vi "Log in with Email and Password.vi"() -> ()   [LabVIEW 2022 SP3]
uses:
  firebase.lvclass
panel:
  out "firebase out":refnum<class "firebase.lvclass">
  in  "Email":string
  in  "Password":string
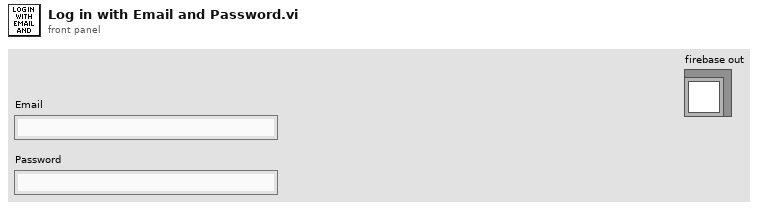
[diagram p1: front panel]
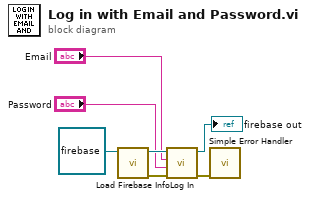
[diagram p0: block diagram]
diagram:
  n1 = call "Load Firebase Info.vi"("firebase in"=refnum<class "firebase.lvclass"> refnum ("firebase.lvclass")) -> ("error out"=w7:errorcluster, "firebase out"=w4:refnum<class "firebase.lvclass">)  [unwired: 9 in]
  n2 = call-dynamic "Log In.vi"("error in"=w7, "password"="Password", "email"="Email", "firebase in"=w4) -> ("error out"=w6:errorcluster, "firebase out"=→"firebase out":refnum<class "firebase.lvclass">)  [unwired: 6 in]
  n3 = call <vilib>:"Simple Error Handler.vi"("error in (no error)"=w6) -> ()  [unwired: 4 in, 5 out]
